vi "Git_Commit.vi"(8 "error in (no error)":errorcluster caption="entrée d'erreur (pas d'erreur)", 10 "Message":string, 11 "Chemin in":path) -> (0 "error out":errorcluster caption="sortie d'erreur", 3 "Chemin out":path)   [LabVIEW 2021]
uses:
  <userlib>/_OpenG.lib/file/file.llb/File Exists - Scalar__ogtk.vi
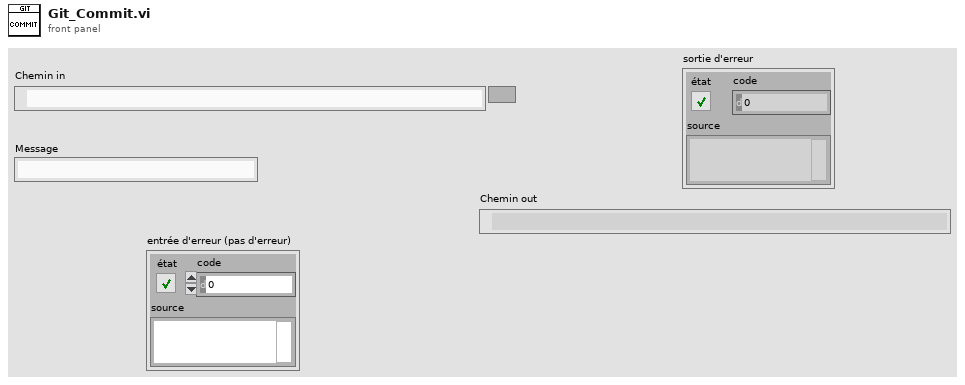
[diagram p1: front panel]
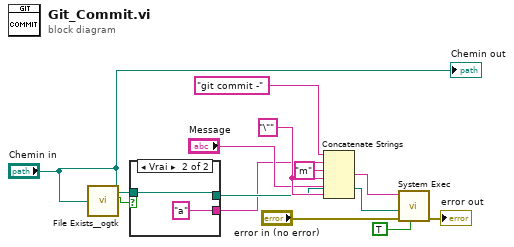
[diagram p0: block diagram]
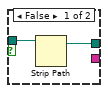
[diagram p2: hidden frame]
diagram:
  w10 = "\"" ("chaîne")
  n1 = call-poly <userlib>:"File Exists__ogtk.vi"("file path"="Chemin in") -> ("is directory"=w3:bool)  [unwired: 6 in, 1 out]
  n2 = case shown="Vrai" w3 {
    tunnel: [w14 w16] -> w6
    tunnel: "Chemin in" -> [w13 w16]
    tunnel: [_ "a"] -> w2
    frame False {
      n3 = Strip Path(path=w13) -> (stripped path=w14:path)  [unwired: 1 out]
    }
    frame True {
    }
  }
  n4 = Concatenate Strings("git commit -", w2, "m" ("chaîne"), w10, "Message", w10) -> (w11:string)
  n5 = call <vilib>:"System Exec.vi"("run minimized? (F)"=TRUE, "error in (no error)"="error in (no error)", "working directory"=w6, "command line"=w11) -> ("error out"=→"error out":errorcluster)  [unwired: 4 in, 3 out]
  "Chemin out" <- "Chemin in"
